vi "GetParam.vi"(8 "error in (no error)":errorcluster caption="entrée d'erreur (pas d'erreur)", 11 "Classification_Report.lvclass":refnum<class "Classification_Report.lvclass">) -> (0 "error out":errorcluster caption="sortie d'erreur", 2 "classification_report":T1={"labels"=[], "target_names"=[], "sample_weight"=[], "digits"=2, "zero_division"={"dtype_zero_division"="str", "zero_division"="warn"}}, 3 "Classification_Report.lvclass":refnum<class "Classification_Report.lvclass">)   [LabVIEW 2020, in "Classification_Report.lvclass"]
doc: "Get Parameters"
uses:
  Classification_Report.lvclass
  Classification_Report.lvclass/Classification_Report.ctl
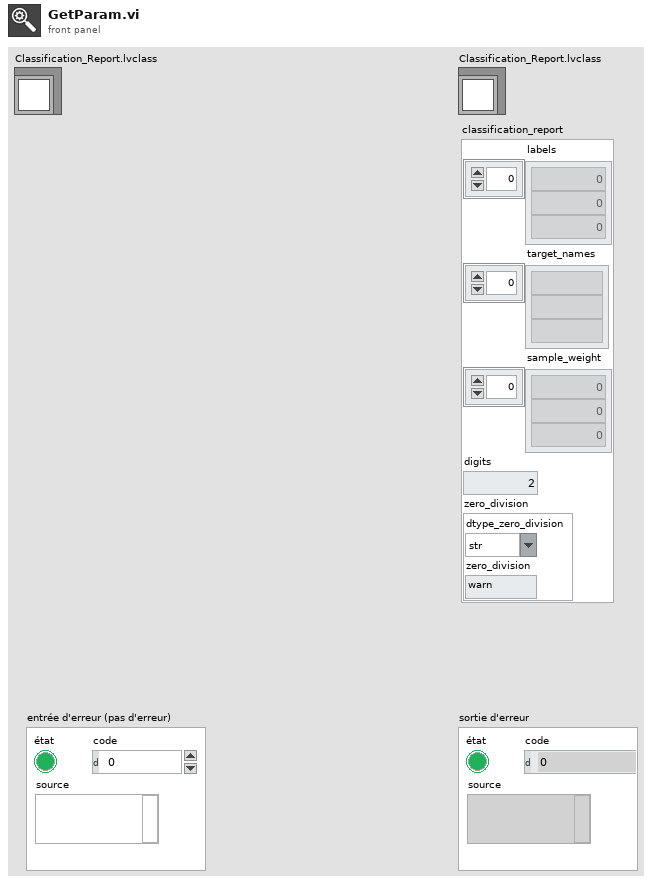
[diagram p1: front panel]
types:
  T1 = cluster{"labels":i32[], "target_names":string[], "sample_weight":dbl[], "digits":i32, "zero_division":cluster{"dtype_zero_division":string, "zero_division":string}}
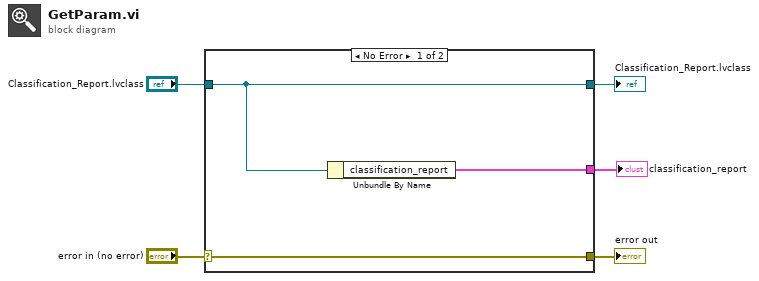
[diagram p0: block diagram]
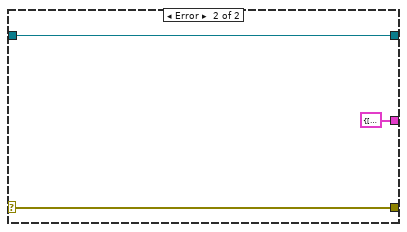
[diagram p2: hidden frame]
diagram:
  n1 = case shown="No Error" "error in (no error)" {
    selector: "error in (no error)" -> [w8 w10]
    tunnel: [w8 w10] -> w4
    tunnel: [w7 w11] -> w2
    tunnel: "Classification_Report.lvclass" -> [w7 w11]
    tunnel: [w6 T1 {"labels"=[], "target_names"=[], "sample_weight"=[], "digits"=0, "zero_division"={"dtype_zero_division"="", "zero_division"=""}} ("classification_report")] -> w1
    frame No Error {
      n2 = Unbundle By Name(w7) -> ("classification_report"=w6:T1)
    }
    frame Error {
    }
  }
  "error out" <- w4
  "Classification_Report.lvclass" <- w2
  "classification_report" <- w1
